vi "Set Path Tag.vi"(8 "error in (no error)":errorcluster, 9 "Tag Value":string, 10 "Tag Name":string, 11 "Log File Specification in":refnum<class "Log File Specification.lvclass">) -> (0 "error out":errorcluster, 3 "Log File Specification out":refnum<class "Log File Specification.lvclass">)   [LabVIEW 2012, in "Waveform Data Logger Shared.lvlib" / "Log File Specification.lvclass"]
uses:
  Log File Specification.lvclass
  Log File Specification.lvclass/Log File Specification.ctl
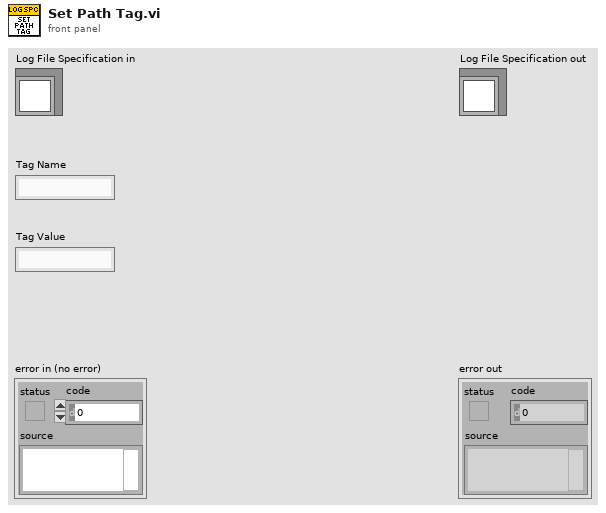
[diagram p1: front panel]
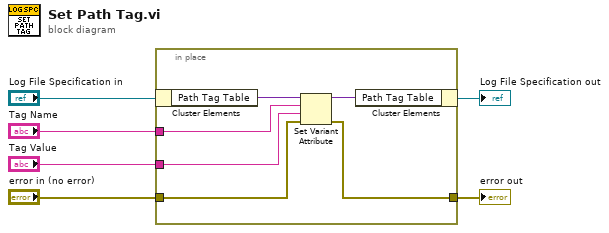
[diagram p0: block diagram]
diagram:
  n1 = in-place {
    in-place-border: "error in (no error)" -> [w10]
    in-place-border: [w9] -> w3
    in-place-border: "Tag Name" -> [w8]
    in-place-border: "Tag Value" -> [w7]
    n2 = in-place-cluster #1("Log File Specification in") -> ("Path Tag Table"=w12:variant)
    n3 = Set Variant Attribute(Variant=w12, name=w8, value=w7, error in=w10) -> (Variant out=w11:variant, error out=w9:errorcluster)  [unwired: 1 out]
    n4 = in-place-cluster #1("Path Tag Table"=w11) -> (→"Log File Specification out":refnum<class "Log File Specification.lvclass">)
  }
  "error out" <- w3
